vi "Init & Start Auto Refresh.vi"(8 "error in (no error)":errorcluster, 9 "Channel Mask":u64, 10 "Config Data":T2, 11 "Connection Data In":T1) -> (0 "error out":errorcluster, 3 "Connection Data Out":T1)   [LabVIEW 2014, in "MSX-E3711_dll.lvlib"]
doc: "Toma los datos de configuracion y su dll se encarga de pasarle los parametros al ADDI-DATA."
uses:
  MSX-E3711_dll.lvlib
  Typedef/Config Data.ctl
  Typedef/Connection Data.ctl
  E:/Repositorio Magnis/INF002/v0/Modules/HAL/Drivers/Sync/ADDI-DATA MSX-E3711/API/MSXE371x.dll
  MSXE371x.dll
  E:/Repositorio Magnis/INF002/v0/Modules/HAL/Drivers/Sync/ADDI-DATA MSX-E3711/API/MXCommon.dll
  MXCommon.dll
panel:
  out "Status Autorefresh":string="Success."
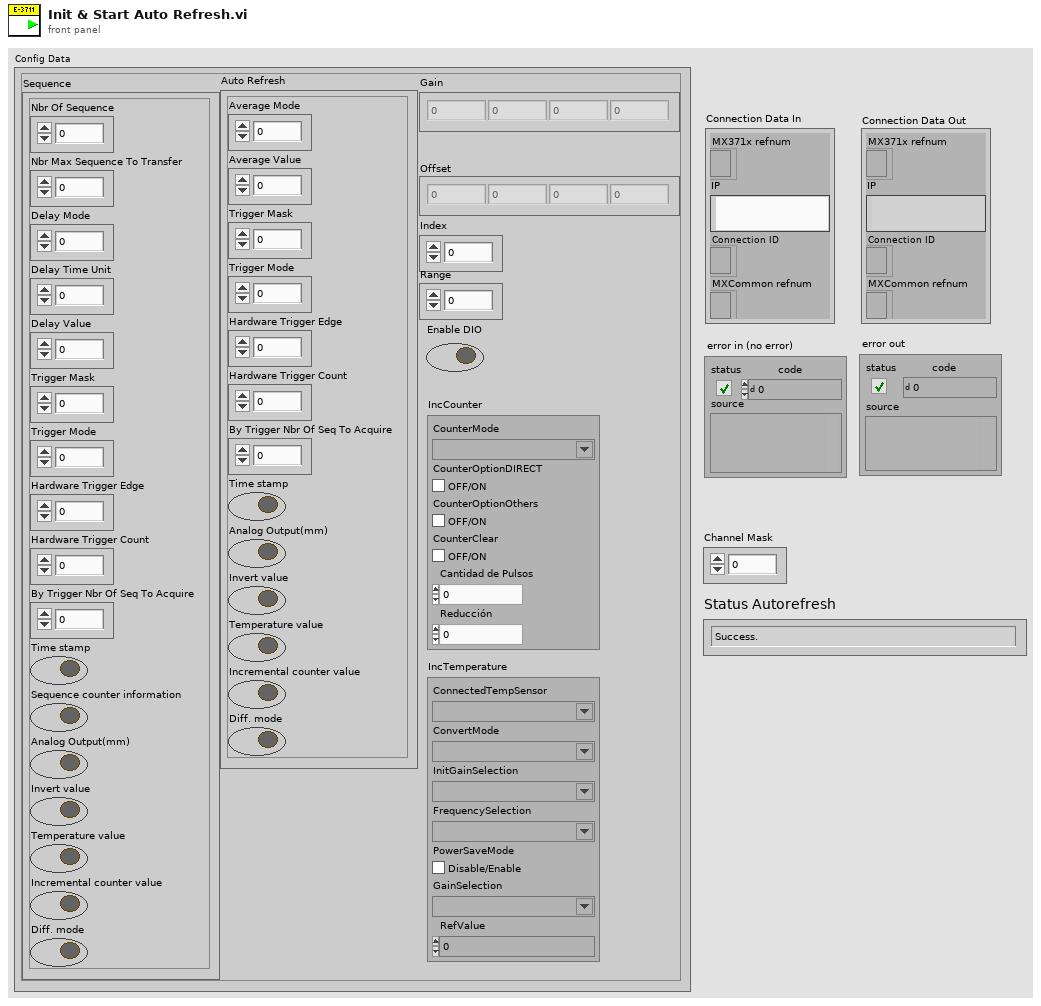
[diagram p1: front panel]
types:
  T1 = typedef "MSX-E3711_dll.lvlib/Connection Data.ctl" = cluster{"MX371x refnum":refnum<k24>, "IP":string, "Connection ID ":refnum<k5>, "MXCommon refnum":refnum<k24>}
  T2 = typedef "MSX-E3711_dll.lvlib/Config Data.ctl" = cluster{"Auto Refresh":cluster{"Average Mode":u64, "Average Value":u64, "Trigger Mask":u64, "Trigger Mode":u64, "Hardware Trigger Edge":u64, "Hardware Trigger Count":u64, "By Trigger Nbr Of Seq To Acquire":u64, "Time stamp":bool, "Analog Output(mm)":bool, "Invert value":bool, "Temperature value":bool, "Incremental counter value":bool, "Diff. mode":bool}, "Gain":sgl[], "Offset":sgl[], "Index":u64, "Range":sgl, "Sequence":cluster{"Nbr Of Sequence":u64, "Nbr Max Sequence To Transfer":u64, "Delay Mode":u64, "Delay Time Unit":u64, "Delay Value":u64, "Trigger Mask":u64, "Trigger Mode":u64, "Hardware Trigger Edge":u64, "Hardware Trigger Count":u64, "By Trigger Nbr Of Seq To Acquire":u64, "Time stamp":bool, "Sequence counter information":bool, "Analog Output(mm)":bool, "Invert value":bool, "Temperature value":bool, "Incremental counter value":bool, "Diff. mode":bool}, "Enable DIO":bool, "IncCounter":cluster{"CounterMode":string, "CounterOptionDIRECT  ":bool, "CounterOptionOthers":bool, "CounterClear ":bool, "Cantidad de Pulsos":sgl, "Reducción":sgl}, "IncTemperature":cluster{"ConnectedTempSensor":string, "ConvertMode":string, "InitGainSelection":string, "FrequencySelection":string, "PowerSaveMode":bool, "GainSelection":string, "RefValue":dbl}}
  T3 = cluster{"Average Mode":u64, "Average Value":u64, "Trigger Mask":u64, "Trigger Mode":u64, "Hardware Trigger Edge":u64, "Hardware Trigger Count":u64, "By Trigger Nbr Of Seq To Acquire":u64, "Time stamp":bool, "Analog Output(mm)":bool, "Invert value":bool, "Temperature value":bool, "Incremental counter value":bool, "Diff. mode":bool}
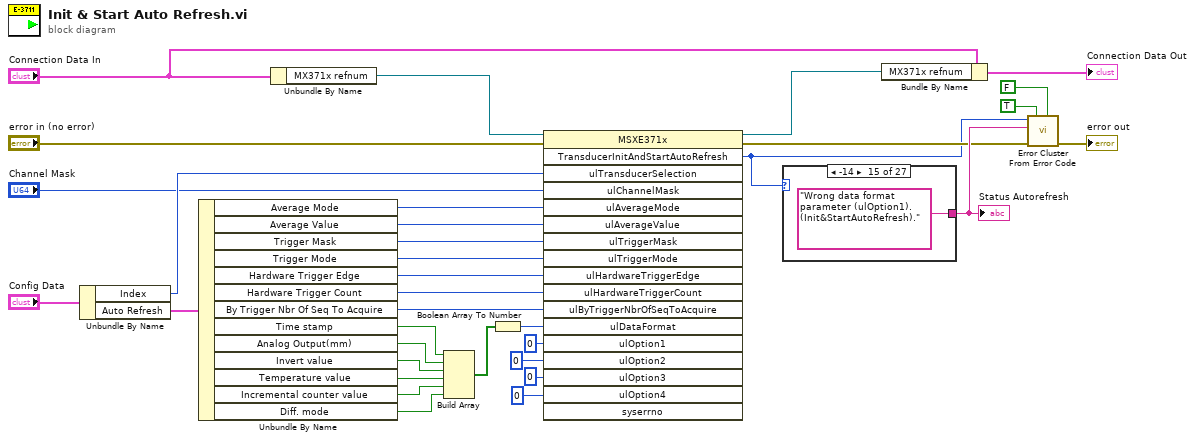
[diagram p0: block diagram]
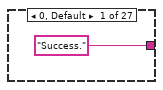
[diagram p2: hidden frame]
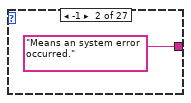
[diagram p3: hidden frame]
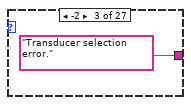
[diagram p4: hidden frame]
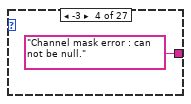
[diagram p5: hidden frame]
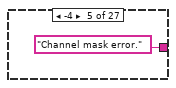
[diagram p6: hidden frame]
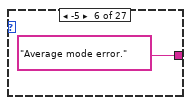
[diagram p7: hidden frame]
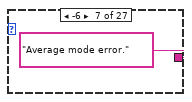
[diagram p8: hidden frame]
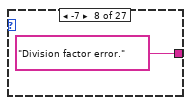
[diagram p9: hidden frame]
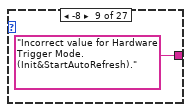
[diagram p10: hidden frame]
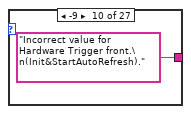
[diagram p11: hidden frame]
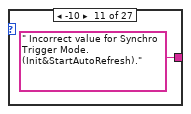
[diagram p12: hidden frame]
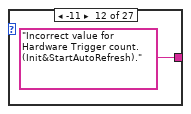
[diagram p13: hidden frame]
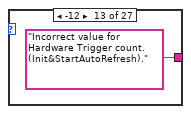
[diagram p14: hidden frame]
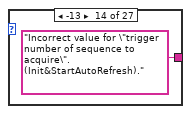
[diagram p15: hidden frame]
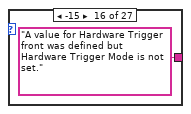
[diagram p16: hidden frame]
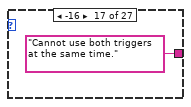
[diagram p17: hidden frame]
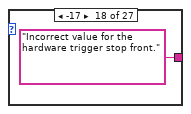
[diagram p18: hidden frame]
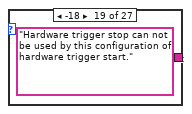
[diagram p19: hidden frame]
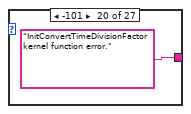
[diagram p20: hidden frame]
diagram:
  n1 = Unbundle By Name("Config Data") -> ("Index"=w17:u64, "Auto Refresh"=w34:T3)
  n2 = Unbundle By Name(w34) -> ("Average Mode"=w12:u64, "Average Value"=w11:u64, "Trigger Mask"=w10:u64, "Trigger Mode"=w9:u64, "Hardware Trigger Edge"=w8:u64, "Hardware Trigger Count"=w7:u64, "By Trigger Nbr Of Seq To Acquire"=w6:u64, "Time stamp"=w33:bool, "Analog Output(mm)"=w31:bool, "Invert value"=w32:bool, "Temperature value"=w22:bool, "Incremental counter value"=w21:bool, "Diff. mode"=w23:bool)
  n3 = Unbundle By Name("Connection Data In") -> ("MX371x refnum"=w20:refnum<k24>)
  n4 = Build Array(w33, w31, w32, w22, w21, w23) -> (w30:bool[])
  n5 = Boolean Array To Number(Boolean array=w30) -> (number=w14:u32)
  n6 = invoke class="MSXE371x" method="TransducerInitAndStartAutoRefresh"(reference=w20, error in="error in (no error)", "ulTransducerSelection"=w17, "ulChannelMask"="Channel Mask", "ulAverageMode"=w12, "ulAverageValue"=w11, "ulTriggerMask"=w10, "ulTriggerMode"=w9, "ulHardwareTriggerEdge"=w8, "ulHardwareTriggerCount"=w7, "ulByTriggerNbrOfSeqToAcquire"=w6, "ulDataFormat"=w14, "ulOption1"=u64 0 ("ulOption2"), "ulOption2"=u64 0 ("ulOption3"), "ulOption3"=u64 0 ("ulOption4"), "ulOption4"=u64 0 ("ulOption3")) -> (reference out=w19:refnum<k24>, error out=w18:errorcluster, "TransducerInitAndStartAutoRefresh"=w16:i32)  [unwired: 2 in, 15 out]
  n7 = case shown="-14" w16 {
    tunnel: ["Success." "Means an system error occurred." "Transducer selection error." "Channel mask error : can not be null." "Channel mask error." "Average mode error." "Average mode error." "Division factor error." "Incorrect value for Hardware Trigger Mode. (Init&StartAutoRefresh)." "Incorrect value for Hardware Trigger front.\n(Init&StartAutoRefresh)." " Incorrect value for Synchro Trigger Mode. (Init&StartAutoRefresh)." "Incorrect value for Hardware Trigger count. (Init&StartAutoRefresh)." "Incorrect value for Hardware Trigger count. (Init&StartAutoRefresh)." "Incorrect value for \"trigger number of sequence to acquire\". (Init&StartAutoRefresh)." "Wrong data format parameter (ulOption1). (Init&StartAutoRefresh)." "A value for Hardware Trigger front was defined but Hardware Trigger Mode is not set." "Cannot use both triggers at the same time." "Incorrect value for the hardware trigger stop front." "Hardware trigger stop can not be used by this configuration of hardware trigger start." "InitConvertTimeDivisionFactor kernel function error." "SetAutoRefreshAverageValue kernel function error." "InitEnableDisableHardwareTrigger kernel function error." "InitDigitalInputFilter kernel function error." "SynchroTrigger Init/Enable/Disable kernel function error." "Internal system error occurred. See value of syserrno" "SetTriggerSequenceCount kernel function error." "StartAutoRefresh kernel function error."] -> w27
    frame 0, Default {
    }
    frame -1 {
    }
    frame -2 {
    }
    frame -3 {
    }
    frame -4 {
    }
    frame -5 {
    }
    frame -6 {
    }
    frame -7 {
    }
    frame -8 {
    }
    frame -9 {
    }
    frame -10 {
    }
    frame -11 {
    }
    frame -12 {
    }
    frame -13 {
    }
    frame -14 {
    }
    frame -15 {
    }
    frame -16 {
    }
    frame -17 {
    }
    frame -18 {
    }
    frame -101 {
    }
    frame -102 {
    }
    frame -104 {
    }
    frame -103 {
    }
    frame -105 {
    }
    frame -100 {
    }
    frame -106 {
    }
    frame -107 {
    }
  }
  "Status Autorefresh" <- w27
  n8 = Bundle By Name(cluster="Connection Data In", "MX371x refnum"=w19) -> (→"Connection Data Out":T1)
  n9 = call <vilib>:"Error Cluster From Error Code.vi"("is warning? (False)"=FALSE, "show call chain? (False)"=TRUE, "error in (no error)"=w18, "error message (\"\")"=w27, "error code (0)"=w16) -> ("error out"=→"error out":errorcluster)  [unwired: 4 in]
